vi "john testing.vi"() -> ()   [LabVIEW 2017, in "Synapse CCD.lvclass"]
uses:
  Synapse CCD.lvclass
  Areas.ctl
  Synapse CCD.lvclass/Synapse CCD.ctl
panel:
  out "ReadCommSetting":variant
  out "where am i?":string
  out "fake check status: populate fields with member data: CCD private data":T2={"JYCCDLib.IJYCCDReqd"=refnum, "JYMONOLib.IJYMonoReqd"=refnum, "Integration time"=0.01, "ADC"=0, "GAIN"=0, "Areas"=[[1, 1, 1, 1024, 256, 1, 256]], "Most Recent Data Object"=refnum, "Mono Properties"={"Grating"=0, "Center Wavelength"=0.0, "Entrance Slit"=0.0, "Exit Slit"=0.0}, "Coverage"={"Max"=0.0, "Min"=0.0}, "Multi-Acquisitions"={"Dark Subtract?"=FALSE, "Averaging?"=FALSE, "Cosmic Ray Removal?"=FALSE, "# to Average"=0, "Time Between Acq."=0, "Acquisitions Control Array"=[TRUE], "Raw Data"=[], "Processed Data"=[], "Array of Wavelengths"=[]}} {"Mono Properties"."Grating" items=["1200 lines/mm - 500 nm Blaze", "1200 lines/mm - 750 nm Blaze", "600 lines/mm - 1000 nm Blaze"]; "GAIN" items=["High Light", "Best Dynamic", "High Sensitivity"]; "ADC" items=["   20 kHz", "1 MHz", "1 MHz Ultra"]}
  out "Synapse CCD out":refnum<class "Synapse CCD.lvclass">
  out "error out":errorcluster
  out "real check status: populate fields with member data: CCD private data":T2={"JYCCDLib.IJYCCDReqd"=refnum, "JYMONOLib.IJYMonoReqd"=refnum, "Integration time"=0.01, "ADC"=0, "GAIN"=0, "Areas"=[[1, 1, 1, 1024, 256, 1, 256]], "Most Recent Data Object"=refnum, "Mono Properties"={"Grating"=0, "Center Wavelength"=0.0, "Entrance Slit"=0.0, "Exit Slit"=0.0}, "Coverage"={"Max"=0.0, "Min"=0.0}, "Multi-Acquisitions"={"Dark Subtract?"=FALSE, "Averaging?"=FALSE, "Cosmic Ray Removal?"=FALSE, "# to Average"=0, "Time Between Acq."=0, "Acquisitions Control Array"=[TRUE], "Raw Data"=[], "Processed Data"=[], "Array of Wavelengths"=[]}} {"Mono Properties"."Grating" items=["1200 lines/mm - 500 nm Blaze", "1200 lines/mm - 750 nm Blaze", "600 lines/mm - 1000 nm Blaze"]; "GAIN" items=["High Light", "Best Dynamic", "High Sensitivity"]; "ADC" items=["   20 kHz", "1 MHz", "1 MHz Ultra"]}
  out "resolution":dbl
  out "end":dbl
  out "start":dbl
  in  "fake wavelength":dbl
  out "Current WL":dbl
  in  "Shutter":bool
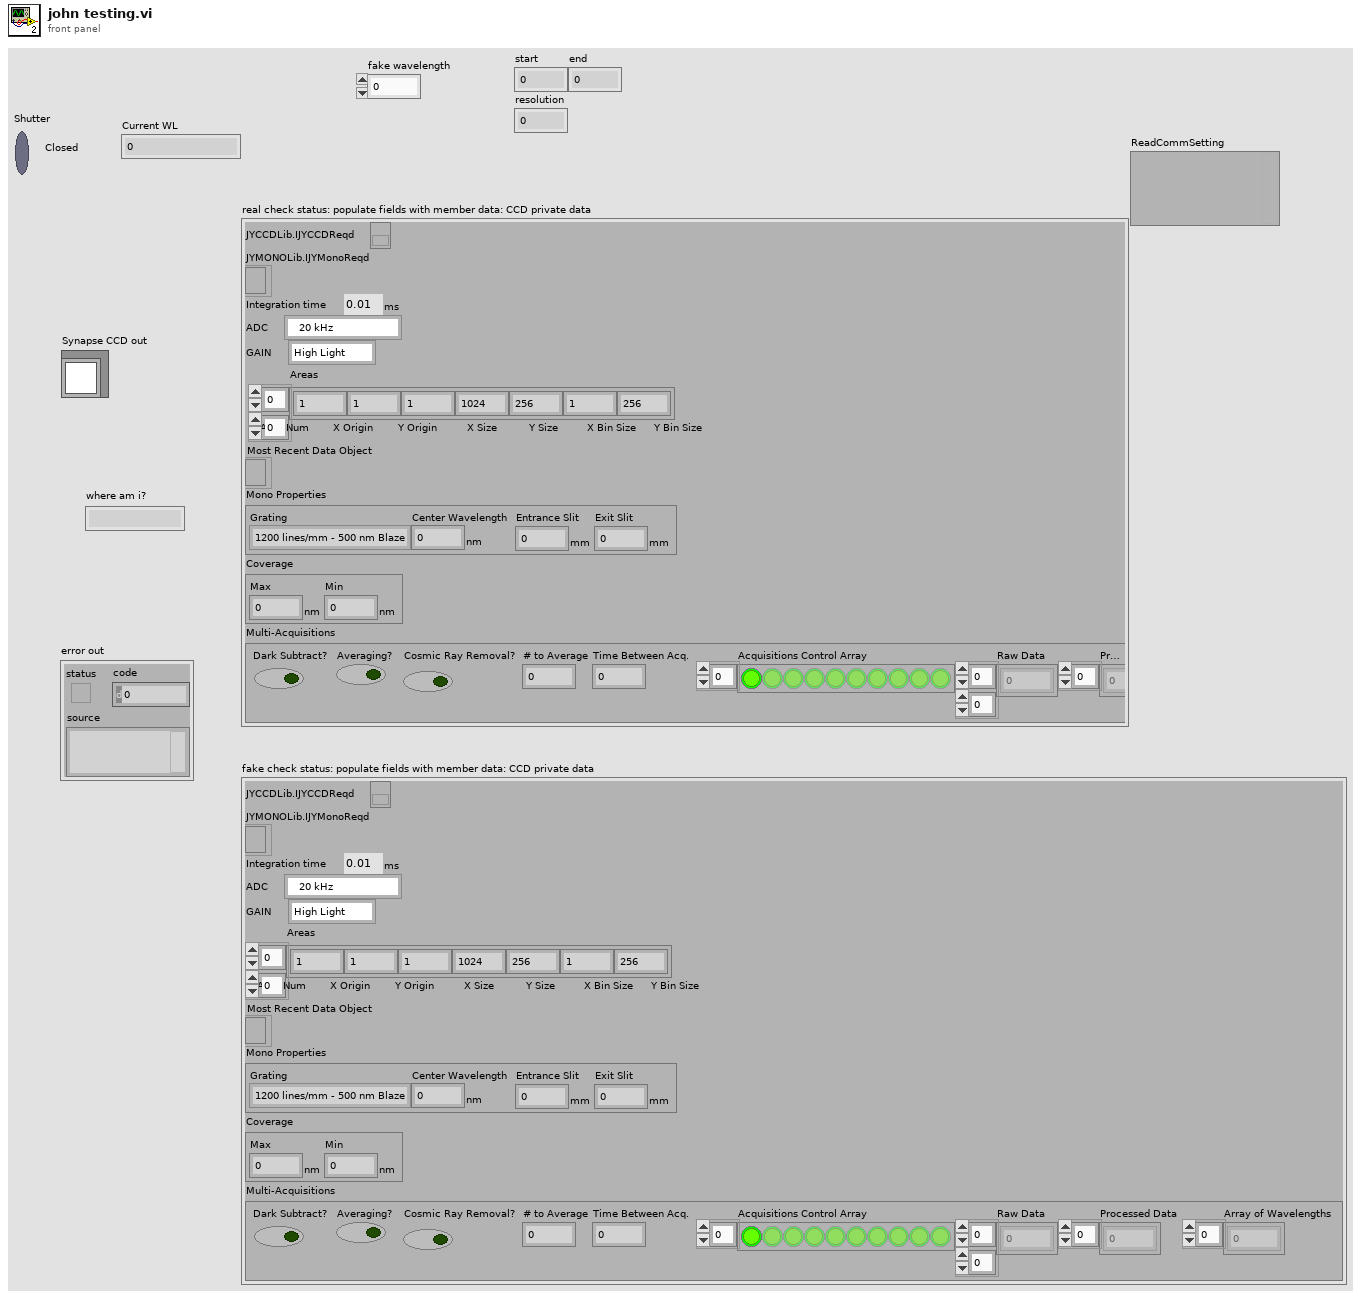
[diagram p1: front panel]
types:
  T1 = typedef "Synapse CCD.lvclass/Areas.ctl" = i32[][]
  T2 = cluster{"JYCCDLib.IJYCCDReqd":refnum<k7>, "JYMONOLib.IJYMonoReqd":refnum<k7>, "Integration time":dbl[unit], "ADC":u16, "GAIN":u16, "Areas":T1, "Most Recent Data Object":refnum<k7>, "Mono Properties":cluster{"Grating":u16, "Center Wavelength":dbl[unit], "Entrance Slit":dbl[unit], "Exit Slit":dbl[unit]}, "Coverage":cluster{"Max":dbl[unit], "Min":dbl[unit]}, "Multi-Acquisitions":cluster{"Dark Subtract?":bool, "Averaging?":bool, "Cosmic Ray Removal?":bool, "# to Average":u32, "Time Between Acq.":u32, "Acquisitions Control Array":bool[], "Raw Data":i32[][], "Processed Data":dbl[], "Array of Wavelengths":dbl[]}}
  T3 = cluster{"Grating":u16, "Center Wavelength":dbl[unit], "Entrance Slit":dbl[unit], "Exit Slit":dbl[unit]}
  T4 = cluster{"Dark Subtract?":bool, "Averaging?":bool, "Cosmic Ray Removal?":bool, "# to Average":u32, "Time Between Acq.":u32, "Acquisitions Control Array":bool[], "Raw Data":i32[][], "Processed Data":dbl[], "Array of Wavelengths":dbl[]}
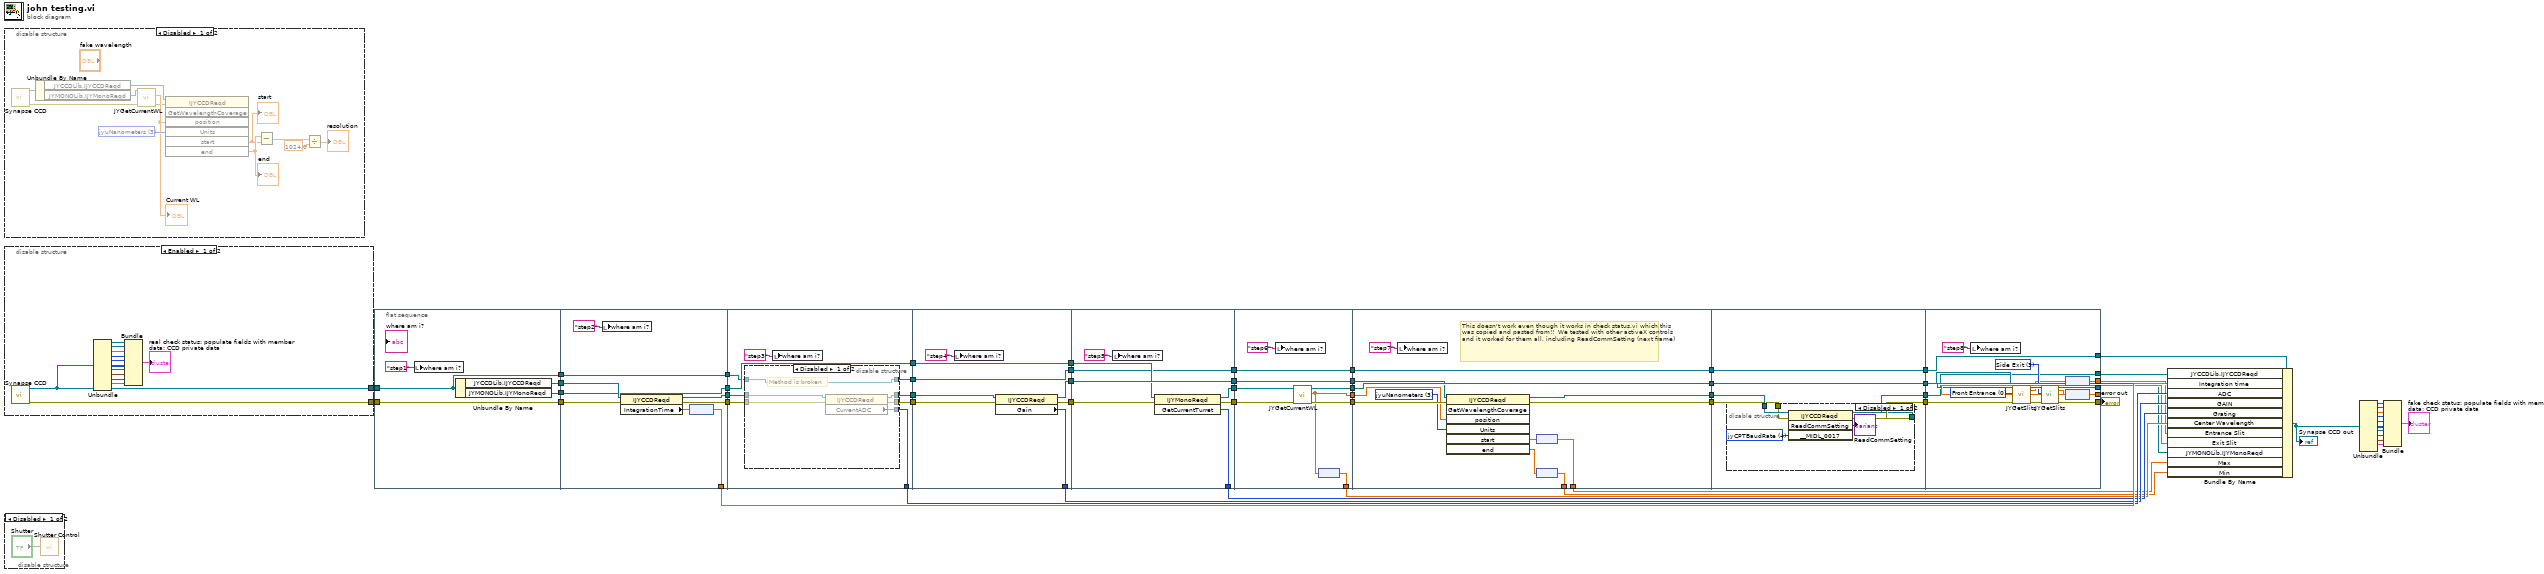
[diagram p0: block diagram]
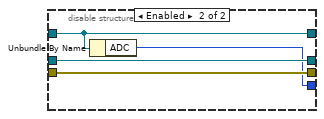
[diagram p2: hidden frame]
diagram:
  n1 = disable-structure shown="Disabled" {
    frame Disabled {
      w72 = 3 items=["jyuUndefined", "jyuMillimeters", "jyuMicrons", "jyuNanometers", "jyuAngstroms", "jyuPicometers", "jyuBandpass", "jyuSteps", "jyuWavenumbers", "jyuDeltaWavenumbers", "jyuElectronVolts", "jyuNanoseconds", "jyuMicroseconds", "jyuMilliseconds", "jyuSeconds", "jyuMinutes", "jyuHours", "jyuVolts", "jyuMillivolts", "jyuMicrovolts", "jyuAmperes", "jyuMilliAmps", "jyuMicroAmps", "jyuCounts", "jyuCountsPerSecond", "jyuDegreesCelcius", "jyuDegreesFahrenheit", "jyuDegreesKelvin", "jyuPixels", "jyuTotalUnitsPlusOne"] ("Units")
      n2 = call "Synapse CCD.vi"() -> ("error out"=w63:errorcluster, "Synapse CCD.lvclass"=w65:refnum<class "Synapse CCD.lvclass">)  [unwired: 10 in]
      n3 = Unbundle By Name(w65) -> ("JYCCDLib.IJYCCDReqd"=w61:refnum<k7>, "JYMONOLib.IJYMonoReqd"=w64:refnum<k7>)
      n4 = call "JYGetCurrentWL.vi"("error in (no error)"=w63, "JYMONOLib.IJYMonoReqd In"=w64) -> ("error out"=w62:errorcluster, "Current WL"=w66:dbl)  [unwired: 6 in, 2 out]
      "Current WL" <- w66
      n5 = invoke class="IJYCCDReqd" method="GetWavelengthCoverage"(reference=w61, error in=w62, "position"=w66, "Units"=w72) -> ("start"=w70:dbl, "end"=w71:dbl)  [unwired: 3 in, 5 out]
      "start" <- w70
      "end" <- w71
      n6 = Subtract(x=w71, y=w70) -> (x-y=w69:dbl)
      n7 = Divide(x=w69, y=1024.0) -> (x/y=→"resolution":dbl)
    }
    frame Enabled {
    }
  }
  n8 = disable-structure shown="Enabled" {
    disable-tunnel: [w73 _] -> w49
    disable-tunnel: [w74 _] -> w48
    frame Enabled {
      n9 = call "Synapse CCD.vi"() -> ("error out"=w73:errorcluster, "Synapse CCD.lvclass"=w74:refnum<class "Synapse CCD.lvclass">)  [unwired: 10 in]
      n10 = Unbundle(w74) -> (w85:refnum<k7>, w84:refnum<k7>, w83:dbl[unit], w82:u16, w81:u16, w80:T1, w79:refnum<k7>, w78:T3, w77:cluster{"Max":dbl[unit], "Min":dbl[unit]}, w76:T4)  [unwired: 1 out]
      n11 = Bundle("JYCCDLib.IJYCCDReqd"=w85, "JYMONOLib.IJYMonoReqd"=w84, "Integration time"=w83, "ADC"=w82, "GAIN"=w81, "Areas"=w80, "Most Recent Data Object"=w79, "Mono Properties"=w78, "Coverage"=w77, "Multi-Acquisitions"=w76) -> (→"real check status: populate fields with member data: CCD private data":T2)  [unwired: 1 in]
    }
    frame Disabled {
    }
  }
  n12 = disable-structure shown="Disabled" {
    frame Disabled {
      n13 = call "Shutter Control.vi"("Shutter"="Shutter") -> ()  [unwired: 2 in, 2 out]
    }
    frame Enabled {
    }
  }
  n14 = flat-sequence {
    tunnel: w49 -> [w88]
    tunnel: w48 -> [w87]
    tunnel: [w87] -> w47
    tunnel: [w91] -> w46
    tunnel: [w88] -> w45
    tunnel: [w89] -> w44
    tunnel: [w96] -> w43
    tunnel: w47 -> [w100]
    tunnel: [w100] -> w42
    tunnel: [w97] -> w41
    tunnel: [w98] -> w22
    tunnel: w46 -> [w95]
    tunnel: w45 -> [w94]
    tunnel: [w92] -> w40
    tunnel: w44 -> [w92]
    tunnel: w43 -> [w107]
    tunnel: [w106] -> w39
    tunnel: w42 -> [w101]
    tunnel: [w104] -> w38
    tunnel: w41 -> [w109]
    tunnel: [w108] -> w37
    tunnel: [w105] -> w21
    tunnel: [w102] -> w36
    tunnel: w40 -> [w102]
    tunnel: w39 -> [w126]
    tunnel: w38 -> [w120]
    tunnel: [w120] -> w35
    tunnel: w37 -> [w127]
    tunnel: [w125] -> w20
    tunnel: [w124] -> w34
    tunnel: [w123] -> w33
    tunnel: [w121] -> w32
    tunnel: w36 -> [w121]
    tunnel: w35 -> [w128]
    tunnel: [w134] -> w19
    tunnel: [w128] -> w31
    tunnel: [w135] -> w30
    tunnel: [w133] -> w29
    tunnel: [w131] -> w28
    tunnel: w34 -> [w132]
    tunnel: w33 -> [w131]
    tunnel: w32 -> [w129]
    tunnel: w31 -> [w136]
    tunnel: w30 -> [w144]
    tunnel: w29 -> [w142]
    tunnel: [w139] -> w18
    tunnel: [w136] -> w27
    tunnel: [w143] -> w26
    tunnel: [w141] -> w25
    tunnel: w28 -> [w140]
    tunnel: [w140] -> w24
    tunnel: [w138] -> w23
    tunnel: w27 -> [w147]
    tunnel: [w147] -> w9
    tunnel: w26 -> [w156]
    tunnel: w25 -> [w157]
    tunnel: [w157] -> w7
    tunnel: [w155] -> w5
    tunnel: w24 -> [w154]
    tunnel: [w153] -> w14
    tunnel: [w152] -> w13
    tunnel: w23 -> [w151]
    tunnel: [w145] -> w3
    tunnel: w9 -> [w163]
    tunnel: [w163] -> w8
    tunnel: w7 -> [w162]
    tunnel: [w162] -> w6
    tunnel: w5 -> [w160]
    tunnel: [w159] -> w4
    tunnel: w3 -> [w161]
    tunnel: [w158] -> w2
    tunnel: [w171] -> w11
    tunnel: w8 -> [w171]
    tunnel: w6 -> [w182]
    tunnel: [w177] -> w17
    tunnel: [w176] -> w16
    tunnel: [w175] -> w50
    tunnel: [w174] -> w15
    tunnel: w4 -> [w173]
    tunnel: w2 -> [w170]
    tunnel: [w170] -> w1
    frame #0 {
      n15 = local write "where am i?"("step1" ("where am i? (check status)")) -> ()
      n16 = Unbundle By Name(w87) -> ("JYCCDLib.IJYCCDReqd"=w91:refnum<k7>, "JYMONOLib.IJYMonoReqd"=w89:refnum<k7>)
    }
    frame #1 {
      n17 = local write "where am i?"("step2" ("where am i? (check status)")) -> ()
      n18 = property class="IJYCCDReqd"(reference=w95, error in=w94) -> (reference out=w97:refnum<k7>, error out=w96:errorcluster, "IntegrationTime"=w99:dbl)
      n19 = node(w99) -> (w98:dbl[unit])
    }
    frame #2 {
      n20 = disable-structure shown="Disabled" {
        disable-tunnel: w109 -> [w115 w119]
        disable-tunnel: [w114 w119] -> w108
        disable-tunnel: w107 -> [w113 w118]
        disable-tunnel: [w112 w118] -> w106
        disable-tunnel: [w111 w117] -> w105
        disable-tunnel: w101 -> [w110 w116]
        disable-tunnel: [w110 w116] -> w104
        frame Disabled {
          # "Method is broken"
          n21 = property class="IJYCCDReqd"(reference=w115, error in=w113) -> (reference out=w114:refnum<k7>, error out=w112:errorcluster, "CurrentADC"=w111:i32)
        }
        frame Enabled {
          n22 = Unbundle By Name(w116) -> ("ADC"=w117:u16)
        }
      }
      n23 = local write "where am i?"("step3" ("where am i? (check status)")) -> ()
    }
    frame #3 {
      n24 = local write "where am i?"("step4" ("where am i? (check status)")) -> ()
      n25 = property class="IJYCCDReqd"(reference=w127, error in=w126) -> (reference out=w123:refnum<k7>, error out=w124:errorcluster, "Gain"=w125:i32)
    }
    frame #4 {
      n26 = local write "where am i?"("step5" ("where am i? (check status)")) -> ()
      n27 = invoke class="IJYMonoReqd" method="GetCurrentTurret"(reference=w129, error in=w132) -> (reference out=w133:refnum<k7>, error out=w135:errorcluster, "GetCurrentTurret"=w134:i32)  [unwired: 1 in]
    }
    frame #5 {
      n28 = local write "where am i?"("step6" ("where am i? (check status)")) -> ()
      n29 = call "JYGetCurrentWL.vi"("error in (no error)"=w144, "JYMONOLib.IJYMonoReqd In"=w142) -> ("error out"=w143:errorcluster, "Current WL"=w138:dbl, "JYMONOLib.IJYMonoReqd Out"=w141:refnum<k7>)  [unwired: 6 in, 1 out]
      n30 = node(w138) -> (w139:dbl[unit])
    }
    frame #6 {
      w146 = 3 items=["jyuUndefined", "jyuMillimeters", "jyuMicrons", "jyuNanometers", "jyuAngstroms", "jyuPicometers", "jyuBandpass", "jyuSteps", "jyuWavenumbers", "jyuDeltaWavenumbers", "jyuElectronVolts", "jyuNanoseconds", "jyuMicroseconds", "jyuMilliseconds", "jyuSeconds", "jyuMinutes", "jyuHours", "jyuVolts", "jyuMillivolts", "jyuMicrovolts", "jyuAmperes", "jyuMilliAmps", "jyuMicroAmps", "jyuCounts", "jyuCountsPerSecond", "jyuDegreesCelcius", "jyuDegreesFahrenheit", "jyuDegreesKelvin", "jyuPixels", "jyuTotalUnitsPlusOne"] ("Units")
      # "This doesn't work even though it works in check status.vi which this was copied and pasted from!!  We tested with other activeX controls and it worked for them all, including ReadCommSetting (next frame)"
      n31 = local write "where am i?"("step7" ("where am i? (check status)")) -> ()
      n32 = invoke class="IJYCCDReqd" method="GetWavelengthCoverage"(reference=w154, error in=w156, "position"=w151, "Units"=w146) -> (reference out=w145:refnum<k7>, error out=w155:errorcluster, "start"=w150:dbl, "end"=w149:dbl)  [unwired: 3 in, 3 out]
      n33 = node(w150) -> (w153:dbl[unit])
      n34 = node(w149) -> (w152:dbl[unit])
    }
    frame #7 {
      n35 = disable-structure shown="Disabled" {
        disable-tunnel: w161 -> [w169 _]
        disable-tunnel: w160 -> [w168 _]
        disable-tunnel: [w167 _] -> w159
        disable-tunnel: [w166 _] -> w158
        frame Disabled {
          w165 = 4 items=["jyCPTUndefined", "jyCPTCommType", "jyCPTPortNum", "jyCPTDeviceName", "jyCPTBaudRate", "jyCPTDatabits", "jyCPTParitybits", "jyCPTStopbits"] ("__MIDL_0017")
          n36 = invoke class="IJYCCDReqd" method="ReadCommSetting"(reference=w169, error in=w168, "__MIDL_0017"=w165) -> (reference out=w166:refnum<k7>, error out=w167:errorcluster, "ReadCommSetting"=→"ReadCommSetting":variant)  [unwired: 1 in, 1 out]
        }
        frame Enabled {
        }
      }
    }
    frame #8 {
      w183 = u16 0 items=["Front Entrance", "Side Entrance", "Front Exit", "Side Exit", "First Intermediate", "Second Intermediate"] ("Slit")
      w184 = u16 3 items=["Front Entrance", "Side Entrance", "Front Exit", "Side Exit", "First Intermediate", "Second Intermediate"] ("Slit")
      n37 = local write "where am i?"("step8" ("where am i? (check status)")) -> ()
      n38 = call "JYGetSlits.vi"("MonoRefNum IN"=w182, "Slit"=w183, "error in (no error)"=w173) -> ("MonoRefNum Out"=w179:refnum<k7>, "Slit Width"=w181:dbl, "error out"=w180:errorcluster)  [unwired: 13 in, 1 out]
      n39 = call "JYGetSlits.vi"("MonoRefNum IN"=w179, "Slit"=w184, "error in (no error)"=w180) -> ("MonoRefNum Out"=w174:refnum<k7>, "Slit Width"=w178:dbl, "error out"=w175:errorcluster)  [unwired: 13 in, 1 out]
      n40 = node(w181) -> (w177:dbl[unit])
      n41 = node(w178) -> (w176:dbl[unit])
    }
  }
  n42 = Bundle By Name(cluster=w11, "JYCCDLib.IJYCCDReqd"=w1, "Integration time"=w22, "ADC"=w21, "GAIN"=w20, "Grating"=w19, "Center Wavelength"=w18, "Entrance Slit"=w17, "Exit Slit"=w16, "JYMONOLib.IJYMonoReqd"=w15, "Max"=w14, "Min"=w13) -> (w10:refnum<class "Synapse CCD.lvclass">)
  "Synapse CCD out" <- w10
  n43 = Unbundle(w10) -> (w60:refnum<k7>, w59:refnum<k7>, w58:dbl[unit], w57:u16, w56:u16, w55:T1, w54:refnum<k7>, w53:T3, w52:cluster{"Max":dbl[unit], "Min":dbl[unit]}, w51:T4)  [unwired: 1 out]
  n44 = Bundle("JYCCDLib.IJYCCDReqd"=w60, "JYMONOLib.IJYMonoReqd"=w59, "Integration time"=w58, "ADC"=w57, "GAIN"=w56, "Areas"=w55, "Most Recent Data Object"=w54, "Mono Properties"=w53, "Coverage"=w52, "Multi-Acquisitions"=w51) -> (→"fake check status: populate fields with member data: CCD private data":T2)  [unwired: 1 in]
  "error out" <- w50
